vi "GdsLanguage_UpdateAllControlsOnVI.vi"(0 "Viref/PathToUpdate(If Empty Uses the caller)":variant, 2 "MatchControlLabelName":string="^_", 5 "error in (no error)":errorcluster, 7 "CreateLanguageFile(Use this to create a languageFile)":bool) -> (13 "AllLanguageFile":string, 19 "error out":errorcluster)   [LabVIEW 2020]
doc: "Returns a translated string based on the value of the StringID parameter."
panel:
  out "OnlyNew":string
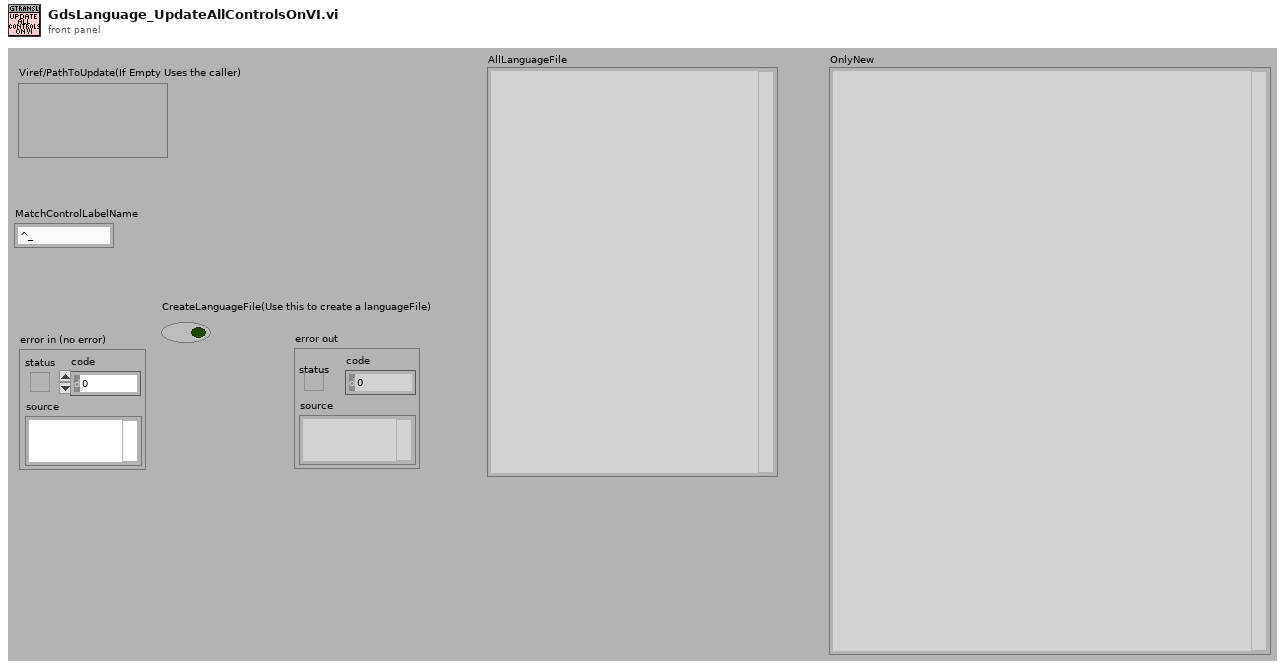
[diagram p1: front panel]
types:
  T1 = cluster{"ViRef":refnum<vi>, "Controls":refnum<vi>[], "RefCreated":bool}
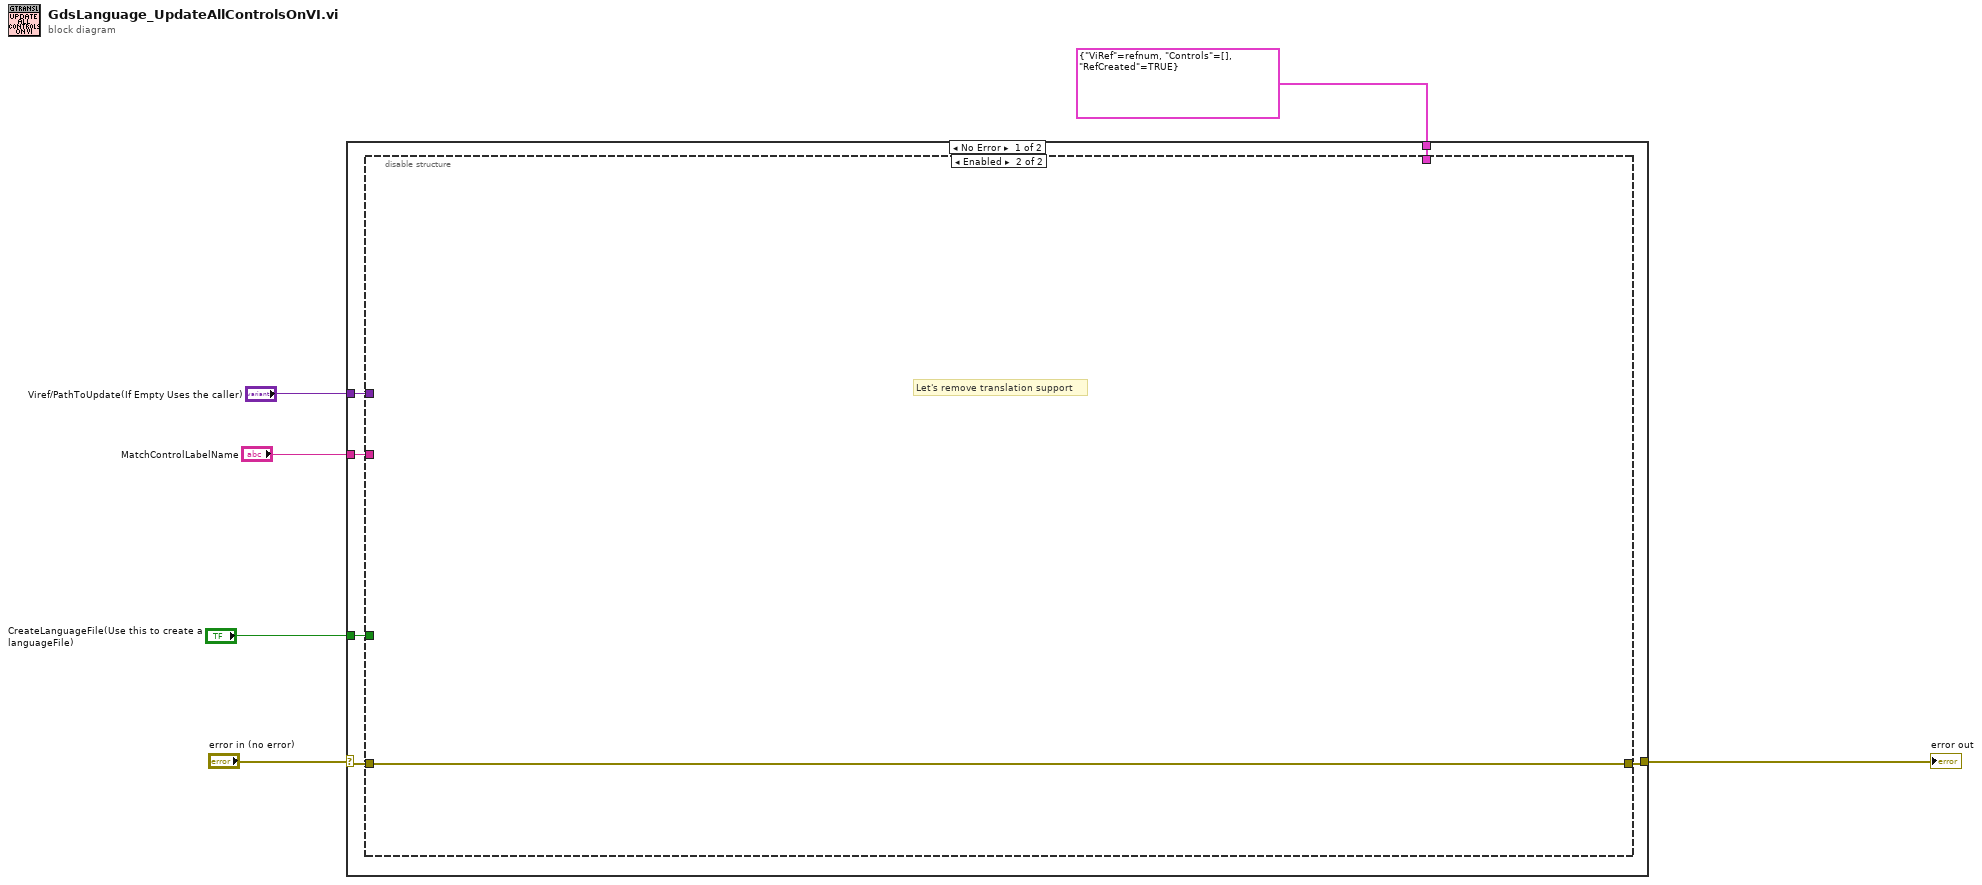
[diagram p0: block diagram]
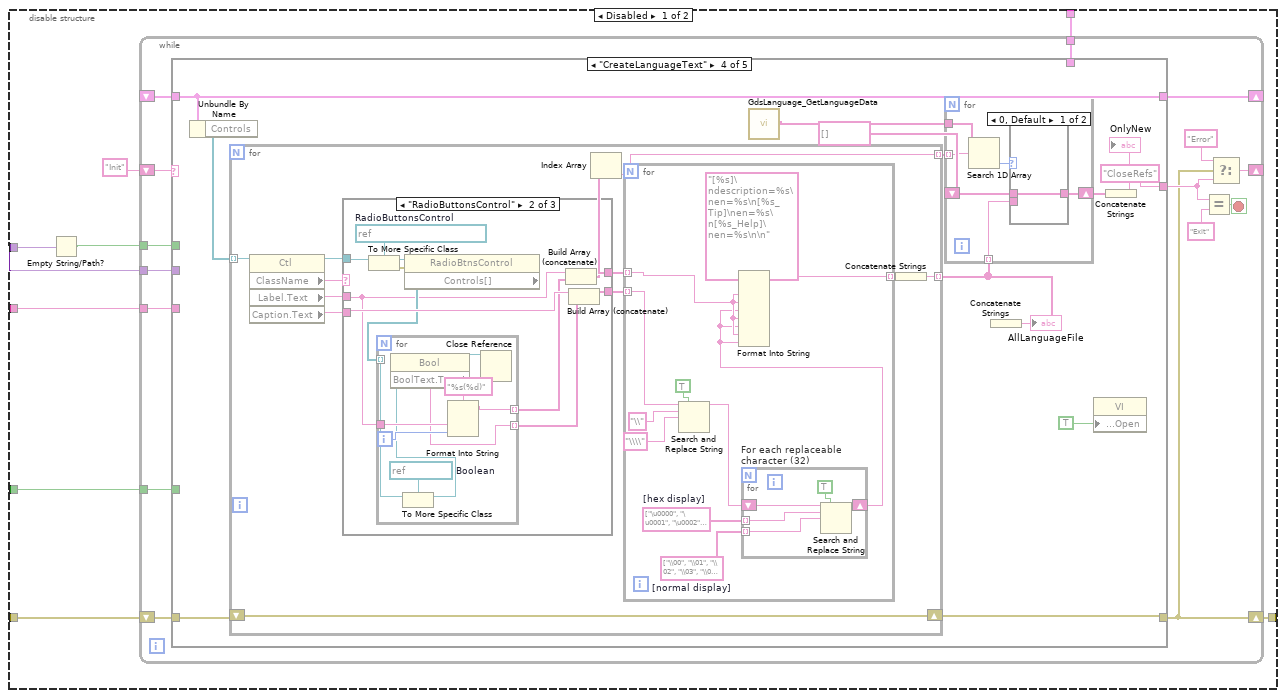
[diagram p2: hidden frame]
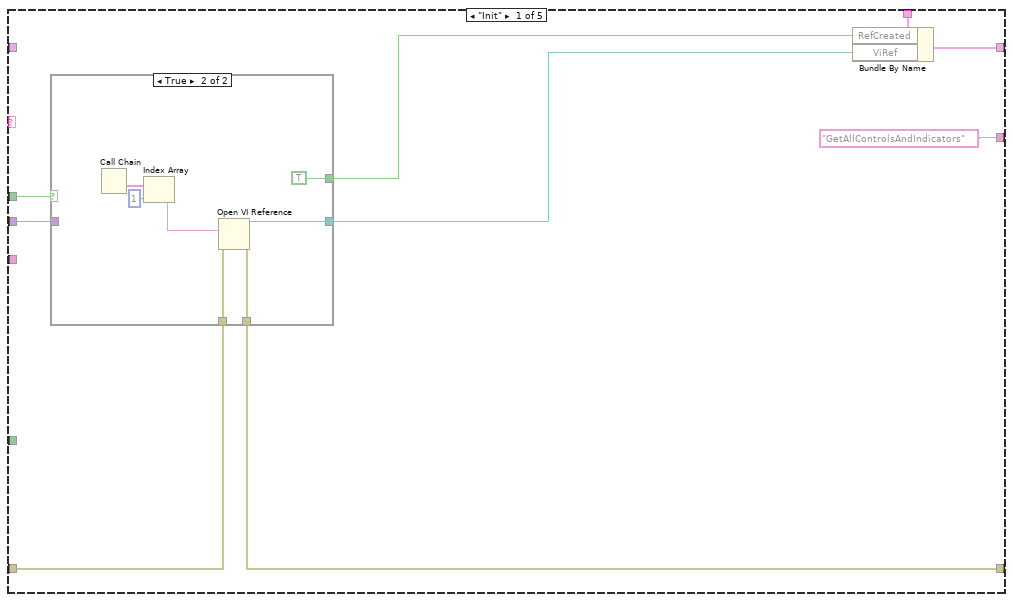
[diagram p3: hidden frame]
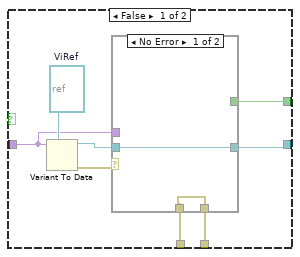
[diagram p4: hidden frame]
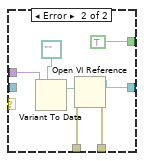
[diagram p5: hidden frame]
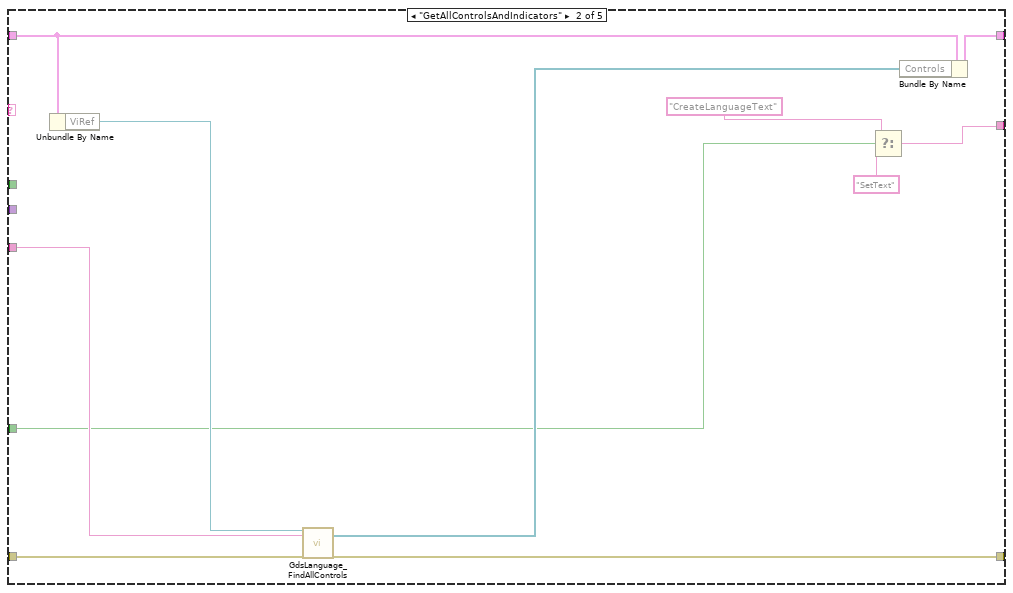
[diagram p6: hidden frame]
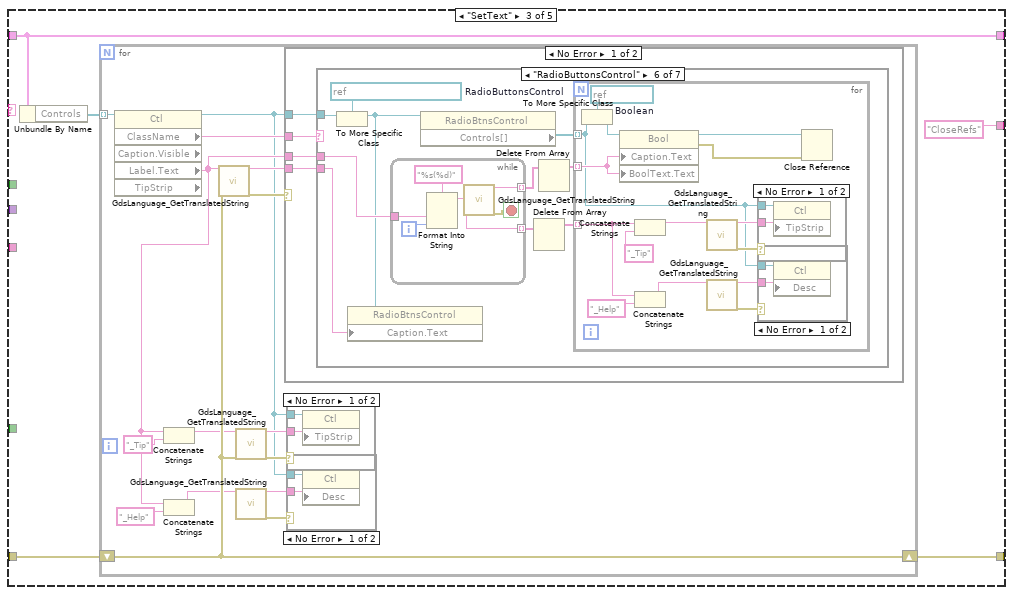
[diagram p7: hidden frame]
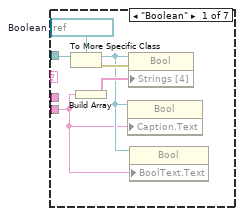
[diagram p10: hidden frame]
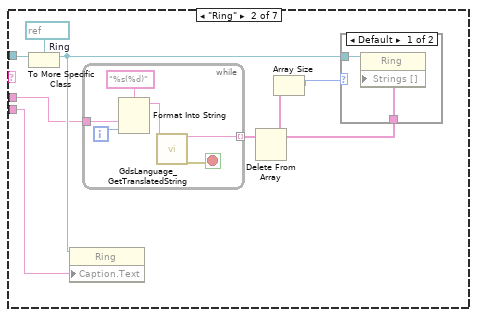
[diagram p11: hidden frame]
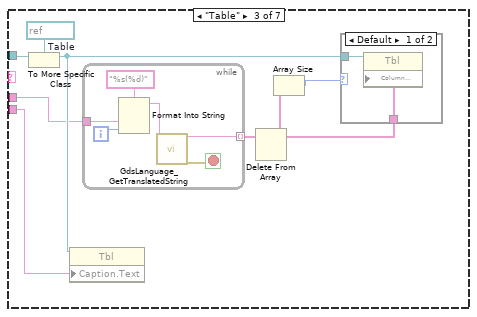
[diagram p13: hidden frame]
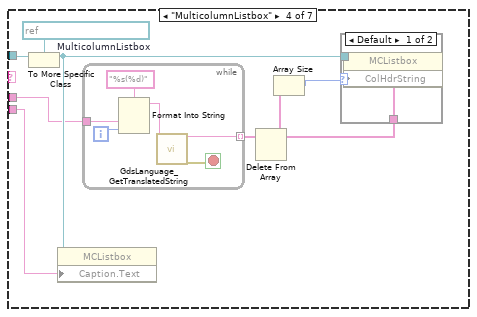
[diagram p15: hidden frame]
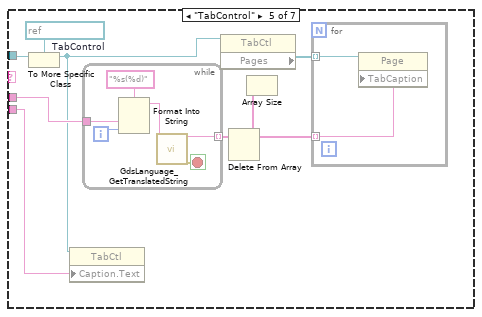
[diagram p17: hidden frame]
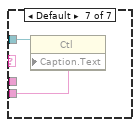
[diagram p20: hidden frame]
diagram:
  n1 = case shown="No Error" "error in (no error)" {
    selector: "error in (no error)" -> [w12 w315]
    tunnel: [w9 w315] -> w5
    tunnel: "Viref/PathToUpdate(If Empty Uses the caller)" -> [w8 _]
    tunnel: "CreateLanguageFile(Use this to create a languageFile)" -> [w7 _]
    tunnel: T1 {"ViRef"=refnum, "Controls"=[], "RefCreated"=TRUE} -> [w11 _]
    tunnel: "MatchControlLabelName" -> [w10 _]
    frame No Error {
      n2 = disable-structure shown="Enabled" {
        disable-tunnel: w12 -> [w19 w314]
        disable-tunnel: w11 -> [w18 _]
        disable-tunnel: w10 -> [w17 _]
        disable-tunnel: [w16 w314] -> w9
        disable-tunnel: w8 -> [w15 _]
        disable-tunnel: w7 -> [w13 _]
        frame Disabled {
          n3 = Empty String/Path?(string/path=w15) -> (empty?=w14:bool)
          n4 = while {
            shift-right: [w28] -> w16
            shift-left: w19 -> [w35]
            shift-right: [w33] -> _
            shift-left: "Init" -> [w34]
            shift-right: [w27] -> _
            shift-left: _ -> [w26]
            tunnel: w14 -> [w25]
            tunnel: w18 -> [w24]
            tunnel: w15 -> [w23]
            tunnel: w17 -> [w22]
            tunnel: w13 -> [w21]
            stop <- w32 stop-if-true
            n5 = case shown="\"CreateLanguageText\"" w34 {
              tunnel: w35 -> [w38 w79 w84 w227 w305]
              tunnel: [w37 w76 w82 w215 w298] -> w28
              tunnel: ["GetAllControlsAndIndicators" w70 "CloseRefs" "CloseRefs" "Exit"] -> w29
              tunnel: [w39 w73 w80 w224 w301] -> w27
              tunnel: w26 -> [_ w75 w80 w224 w301]
              tunnel: w25 -> [w43 _ _ _ _]
              tunnel: w24 -> [w42 _ _ _ _]
              tunnel: w23 -> [w40 _ _ _ _]
              tunnel: w22 -> [_ w78 _ _ _]
              tunnel: w21 -> [_ w72 _ _ w299]
              frame "Init" {
                n6 = case shown="True" w43 {
                  tunnel: w38 -> [w51 w65]
                  tunnel: [w47 w64] -> w41
                  tunnel: w40 -> [w46 _]
                  tunnel: [w50 w63] -> w37
                  tunnel: [w45 TRUE] -> w36
                  frame False {
                    w52 = refnum<vi> refnum  # ViRef
                    n7 = Variant To Data(type=w52, Variant=w46) -> (data=w48:refnum<vi>, error out=w49:errorcluster)  [unwired: 1 in]
                    n8 = case shown="No Error" w49 {
                      tunnel: w51 -> [w53 w61]
                      tunnel: [w53 w60] -> w50
                      tunnel: [w54 w56] -> w47
                      tunnel: w48 -> [w54 _]
                      tunnel: w46 -> [_ w59]
                      tunnel: [_ TRUE] -> w45
                      frame No Error {
                      }
                      frame Error {
                        n9 = Variant To Data(type=path "", Variant=w59) -> (data=w57:path)  [unwired: 1 in, 1 out]
                        n10 = Open VI Reference(vi path=w57, error in (no error)=w61) -> (vi reference=w56:refnum<vi>, error out=w60:errorcluster)  [unwired: 4 in]
                      }
                    }
                  }
                  frame True {
                    n11 = Call Chain() -> (call chain=w68:string[])
                    n12 = Index Array(array=w68, index=1) -> (element=w66:string)
                    n13 = Open VI Reference(vi path=w66, error in (no error)=w65) -> (vi reference=w64:refnum<vi>, error out=w63:errorcluster)  [unwired: 4 in]
                  }
                }
                n14 = Bundle By Name(cluster=w42, "RefCreated"=w36, "ViRef"=w41) -> (w39:T1)
              }
              frame "GetAllControlsAndIndicators" {
                n15 = Unbundle By Name(w75) -> ("ViRef"=w77:refnum<vi>)
                n16 = call <resource>:"GdsLanguage_FindAllControls.vi"("ViRef"=w77, "LabelMatchPattern"=w78, "error in (no error)"=w79) -> ("ControlsFound"=w74:refnum<vi>[], "error out"=w76:errorcluster)  [unwired: 15 in]
                n17 = Select(t="CreateLanguageText", s=w72, f="SetText") -> (s? t:f=w70:string)
                n18 = Bundle By Name(cluster=w75, "Controls"=w74) -> (w73:T1)
              }
              frame "SetText" {
                n19 = Unbundle By Name(w80) -> ("Controls"=w83:refnum<vi>[])
                n20 = for {
                  shift-right: [w95] -> w82
                  shift-left: w84 -> [w95]
                  tunnel: w83 -> [w99] mode=indexing
                  n21 = property class="Ctl" props=["ClassName", "Caption", "Visible", "Label", "Text", "TipStrip"](reference=w99) -> (reference out=w86:refnum<vi>, "ClassName"=w98:string, "Label.Text"=w89:string)  [unwired: 1 in, 3 out]
                  n22 = Concatenate Strings(w89, "_Tip" ("string")) -> (w92:string)
                  n23 = Concatenate Strings(w89, "_Help" ("string")) -> (w85:string)
                  n24 = call <resource>:"GdsLanguage_GetTranslatedString.vi"("StringID(s)"=w89, "error in (no error)"=w95) -> ("FirstStringOut"=w96:string, "error out"=w97:errorcluster)  [unwired: 14 in, 2 out]
                  n25 = call <resource>:"GdsLanguage_GetTranslatedString.vi"("StringID(s)"=w92, "error in (no error)"=w95) -> ("FirstStringOut"=w91:string, "error out"=w94:errorcluster)  [unwired: 14 in, 2 out]
                  n26 = call <resource>:"GdsLanguage_GetTranslatedString.vi"("StringID(s)"=w85) -> ("FirstStringOut"=w88:string, "error out"=w87:errorcluster)  [unwired: 15 in, 2 out]
                  n27 = case shown="No Error" w97 {
                    tunnel: w98 -> [w107 _]
                    tunnel: w86 -> [w105 _]
                    tunnel: w96 -> [w106 _]
                    tunnel: w89 -> [w104 _]
                    frame No Error {
                      n28 = case shown="\"RadioButtonsControl\"" w107 {
                        tunnel: w105 -> [w113 w121 w137 w153 w169 w187 w214]
                        tunnel: w106 -> [w108 w118 w134 w150 w167 w186 w213]
                        tunnel: w104 -> [_ w117 w133 w149 w166 w185 _]
                        frame "Boolean" {
                          w112 = refnum<vi> refnum  # Boolean
                          n29 = To More Specific Class(target class=w112, reference=w113) -> (specific class reference=w109:refnum<vi>, error out=w111:errorcluster)  [unwired: 1 in]
                          n30 = Build Array(w108) -> (w110:string[])
                          n31 = property class="Bool"(reference=w109, "Caption.Text"=w108) -> ()  [unwired: 1 in, 2 out]
                          n32 = property class="Bool"(reference=w109, error in=w111, "Strings [4]"=w110) -> ()  [unwired: 2 out]
                          n33 = property class="Bool"(reference=w109, "BoolText.Text"=w108) -> ()  [unwired: 1 in, 2 out]
                        }
                        frame "Ring" {
                          w120 = refnum<vi> refnum  # Ring
                          n34 = To More Specific Class(target class=w120, reference=w121) -> (specific class reference=w119:refnum<vi>)  [unwired: 1 in, 1 out]
                          n35 = property class="Ring"(reference=w119, "Caption.Text"=w118) -> ()  [unwired: 1 in, 2 out]
                          n36 = while {
                            tunnel: w117 -> [w126]
                            tunnel: [w122] -> w116 mode=indexing
                            i -> [w125]
                            stop <- w123 stop-if-true
                            n37 = Format Into String(format string="%s(%d)", w126, w125) -> (resulting string=w124:string)  [unwired: 2 in, 1 out]
                            n38 = call <resource>:"GdsLanguage_GetTranslatedString.vi"("StringID(s)"=w124) -> ("FirstStringOut"=w122:string, "error out"=w123:errorcluster)  [unwired: 15 in, 2 out]
                          }
                          n39 = Delete From Array(array=w116) -> (array with subset deleted=w114:string[])  [unwired: 2 in, 1 out]
                          n40 = Array Size(array=w114) -> (size(s)=w115:i32)
                          n41 = case shown="Default" w115 {
                            tunnel: w119 -> [w129 _]
                            tunnel: w114 -> [w128 _]
                            frame Default {
                              n42 = property class="Ring"(reference=w129, "Strings []"=w128) -> ()  [unwired: 1 in, 2 out]
                            }
                            frame 0 {
                            }
                          }
                        }
                        frame "Table" {
                          w136 = refnum<vi> refnum  # Table
                          n43 = To More Specific Class(target class=w136, reference=w137) -> (specific class reference=w135:refnum<vi>)  [unwired: 1 in, 1 out]
                          n44 = property class="Tbl"(reference=w135, "Caption.Text"=w134) -> ()  [unwired: 1 in, 2 out]
                          n45 = while {
                            tunnel: w133 -> [w142]
                            tunnel: [w138] -> w132 mode=indexing
                            i -> [w141]
                            stop <- w139 stop-if-true
                            n46 = Format Into String(format string="%s(%d)", w142, w141) -> (resulting string=w140:string)  [unwired: 2 in, 1 out]
                            n47 = call <resource>:"GdsLanguage_GetTranslatedString.vi"("StringID(s)"=w140) -> ("FirstStringOut"=w138:string, "error out"=w139:errorcluster)  [unwired: 15 in, 2 out]
                          }
                          n48 = Delete From Array(array=w132) -> (array with subset deleted=w130:string[])  [unwired: 2 in, 1 out]
                          n49 = Array Size(array=w130) -> (size(s)=w131:i32)
                          n50 = case shown="Default" w131 {
                            tunnel: w135 -> [w145 _]
                            tunnel: w130 -> [w144 _]
                            frame Default {
                              n51 = property class="Tbl"(reference=w145, "Column Headers[]"=w144) -> ()  [unwired: 1 in, 2 out]
                            }
                            frame 0 {
                            }
                          }
                        }
                        frame "MulticolumnListbox" {
                          w152 = refnum<vi> refnum  # MulticolumnListbox
                          n52 = To More Specific Class(target class=w152, reference=w153) -> (specific class reference=w151:refnum<vi>)  [unwired: 1 in, 1 out]
                          n53 = property class="MCListbox"(reference=w151, "Caption.Text"=w150) -> ()  [unwired: 1 in, 2 out]
                          n54 = while {
                            tunnel: w149 -> [w158]
                            tunnel: [w154] -> w148 mode=indexing
                            i -> [w157]
                            stop <- w155 stop-if-true
                            n55 = Format Into String(format string="%s(%d)", w158, w157) -> (resulting string=w156:string)  [unwired: 2 in, 1 out]
                            n56 = call <resource>:"GdsLanguage_GetTranslatedString.vi"("StringID(s)"=w156) -> ("FirstStringOut"=w154:string, "error out"=w155:errorcluster)  [unwired: 15 in, 2 out]
                          }
                          n57 = Delete From Array(array=w148) -> (array with subset deleted=w146:string[])  [unwired: 2 in, 1 out]
                          n58 = Array Size(array=w146) -> (size(s)=w147:i32)
                          n59 = case shown="Default" w147 {
                            tunnel: w151 -> [w161 _]
                            tunnel: w146 -> [w160 _]
                            frame Default {
                              n60 = property class="MCListbox"(reference=w161, "ColHdrString"=w160) -> ()  [unwired: 1 in, 2 out]
                            }
                            frame 0 {
                            }
                          }
                        }
                        frame "TabControl" {
                          w168 = refnum<vi> refnum  # TabControl
                          n61 = To More Specific Class(target class=w168, reference=w169) -> (specific class reference=w163:refnum<vi>)  [unwired: 1 in, 1 out]
                          n62 = property class="TabCtl"(reference=w163, "Caption.Text"=w167) -> ()  [unwired: 1 in, 2 out]
                          n63 = while {
                            tunnel: w166 -> [w176]
                            tunnel: [w172] -> w165 mode=indexing
                            i -> [w175]
                            stop <- w173 stop-if-true
                            n64 = Format Into String(format string="%s(%d)", w176, w175) -> (resulting string=w174:string)  [unwired: 2 in, 1 out]
                            n65 = call <resource>:"GdsLanguage_GetTranslatedString.vi"("StringID(s)"=w174) -> ("FirstStringOut"=w172:string, "error out"=w173:errorcluster)  [unwired: 15 in, 2 out]
                          }
                          n66 = property class="TabCtl"(reference=w163) -> ("Pages"=w162:refnum<vi>[])  [unwired: 1 in, 2 out]
                          n67 = Delete From Array(array=w165) -> (array with subset deleted=w164:string[])  [unwired: 2 in, 1 out]
                          n68 = Array Size(array=w164) -> ()  [unwired: 1 out]
                          n69 = for {
                            tunnel: w164 -> [w171] mode=indexing
                            tunnel: w162 -> [w170] mode=indexing
                            n70 = property class="Page"(reference=w170, "TabCaption"=w171) -> ()  [unwired: 1 in, 2 out]
                          }
                        }
                        frame "RadioButtonsControl" {
                          w180 = refnum<vi> refnum  # RadioButtonsControl
                          n71 = To More Specific Class(target class=w180, reference=w187) -> (specific class reference=w182:refnum<vi>)  [unwired: 1 in, 1 out]
                          n72 = property class="RadioBtnsControl"(reference=w182, "Caption.Text"=w186) -> ()  [unwired: 1 in, 2 out]
                          n73 = while {
                            tunnel: w185 -> [w211]
                            tunnel: [w208] -> w184 mode=indexing
                            tunnel: [w207] -> w179 mode=indexing
                            i -> [w210]
                            stop <- w209 stop-if-true
                            n74 = Format Into String(format string="%s(%d)", w211, w210) -> (resulting string=w207:string)  [unwired: 2 in, 1 out]
                            n75 = call <resource>:"GdsLanguage_GetTranslatedString.vi"("StringID(s)"=w207) -> ("FirstStringOut"=w208:string, "error out"=w209:errorcluster)  [unwired: 15 in, 2 out]
                          }
                          n76 = property class="RadioBtnsControl"(reference=w182) -> ("Controls[]"=w181:refnum<vi>[])  [unwired: 1 in, 2 out]
                          n77 = Delete From Array(array=w179) -> (array with subset deleted=w178:string[])  [unwired: 2 in, 1 out]
                          n78 = Delete From Array(array=w184) -> (array with subset deleted=w183:string[])  [unwired: 2 in, 1 out]
                          n79 = for {
                            tunnel: w183 -> [w196] mode=indexing
                            tunnel: w181 -> [w189] mode=indexing
                            tunnel: w178 -> [w188] mode=indexing
                            w200 = refnum<vi> refnum  # Boolean
                            n80 = To More Specific Class(target class=w200, reference=w189) -> (specific class reference=w199:refnum<vi>)  [unwired: 1 in, 1 out]
                            n81 = property class="Bool"(reference=w199, "Caption.Text"=w196, "BoolText.Text"=w196) -> (reference out=w201:refnum<vi>, error out=w202:errorcluster)  [unwired: 1 in]
                            n82 = Concatenate Strings(w188, "_Tip" ("string")) -> (w191:string)
                            n83 = Concatenate Strings(w188, "_Help" ("string")) -> (w190:string)
                            n84 = call <resource>:"GdsLanguage_GetTranslatedString.vi"("StringID(s)"=w191) -> ("FirstStringOut"=w193:string, "error out"=w192:errorcluster)  [unwired: 15 in, 2 out]
                            n85 = call <resource>:"GdsLanguage_GetTranslatedString.vi"("StringID(s)"=w190) -> ("FirstStringOut"=w194:string, "error out"=w195:errorcluster)  [unwired: 15 in, 2 out]
                            n86 = case shown="No Error" w192 {
                              tunnel: w193 -> [w206 _]
                              tunnel: w189 -> [w205 _]
                              frame No Error {
                                n87 = property class="Ctl"(reference=w205, "TipStrip"=w206) -> ()  [unwired: 1 in, 2 out]
                              }
                              frame Error {
                              }
                            }
                            n88 = case shown="No Error" w195 {
                              tunnel: w194 -> [w204 _]
                              tunnel: w189 -> [w203 _]
                              frame No Error {
                                n89 = property class="Ctl"(reference=w203, "Desc"=w204) -> ()  [unwired: 1 in, 2 out]
                              }
                              frame Error {
                              }
                            }
                            n90 = Close Reference(reference=w201, error in (no error)=w202) -> ()  [unwired: 1 out]
                          }
                        }
                        frame Default {
                          n91 = property class="Ctl"(reference=w214, "Caption.Text"=w213) -> ()  [unwired: 1 in, 2 out]
                        }
                      }
                    }
                    frame Error {
                    }
                  }
                  n92 = case shown="No Error" w94 {
                    tunnel: w91 -> [w103 _]
                    tunnel: w86 -> [w102 _]
                    frame No Error {
                      n93 = property class="Ctl"(reference=w102, "TipStrip"=w103) -> ()  [unwired: 1 in, 2 out]
                    }
                    frame Error {
                    }
                  }
                  n94 = case shown="No Error" w87 {
                    tunnel: w88 -> [w101 _]
                    tunnel: w86 -> [w100 _]
                    frame No Error {
                      n95 = property class="Ctl"(reference=w100, "Desc"=w101) -> ()  [unwired: 1 in, 2 out]
                    }
                    frame Error {
                    }
                  }
                }
              }
              frame "CreateLanguageText" {
                n96 = Unbundle By Name(w224) -> ("Controls"=w226:refnum<vi>[])
                n97 = for {
                  shift-right: [w245] -> w215
                  shift-left: w227 -> [w245]
                  tunnel: w226 -> [w248] mode=indexing
                  tunnel: [w240] -> w219 mode=indexing
                  tunnel: [w238] -> w221 mode=indexing
                  n98 = property class="Ctl"(reference=w248) -> (reference out=w246:refnum<vi>, "ClassName"=w247:string, "Label.Text"=w241:string, "Caption.Text"=w244:string)  [unwired: 1 in, 1 out]
                  n99 = case shown="\"RadioButtonsControl\"" w247 {
                    tunnel: w246 -> [w273 w284 _]
                    tunnel: [w267 w279 w296] -> w242
                    tunnel: w244 -> [_ w278 w297]
                    tunnel: w241 -> [w265 w274 w295]
                    tunnel: [w266 w280 w294] -> w239
                    frame "Boolean" {
                      w272 = refnum<vi> refnum  # Boolean
                      n100 = To More Specific Class(target class=w272, reference=w273) -> (specific class reference=w271:refnum<vi>, error out=w270:errorcluster)  [unwired: 1 in]
                      n101 = property class="Bool"(reference=w271, error in=w270) -> ("Strings [4]"=w269:string[])  [unwired: 2 out]
                      n102 = Index Array(array=w269) -> (element=w268:string)  [unwired: 1 in]
                      n103 = Build Array(w265) -> (w266:string[])
                      n104 = Build Array(w268) -> (w267:string[])
                    }
                    frame "RadioButtonsControl" {
                      w283 = refnum<vi> refnum  # RadioButtonsControl
                      n105 = To More Specific Class(target class=w283, reference=w284) -> (specific class reference=w282:refnum<vi>, error out=w281:errorcluster)  [unwired: 1 in]
                      n106 = property class="RadioBtnsControl"(reference=w282, error in=w281) -> ("Controls[]"=w277:refnum<vi>[])  [unwired: 2 out]
                      n107 = for {
                        tunnel: w277 -> [w286] mode=indexing
                        tunnel: [w290] -> w276 mode=indexing
                        tunnel: [w289] -> w275 mode=indexing
                        tunnel: w274 -> [w291]
                        i -> [w292]
                        w287 = refnum<vi> refnum  # Boolean
                        n108 = To More Specific Class(target class=w287, reference=w286) -> (specific class reference=w285:refnum<vi>)  [unwired: 1 in, 1 out]
                        n109 = property class="Bool"(reference=w285) -> (reference out=w288:refnum<vi>, "BoolText.Text"=w289:string)  [unwired: 1 in, 1 out]
                        n110 = Format Into String(format string="%s(%d)", w291, w292) -> (resulting string=w290:string)  [unwired: 2 in, 1 out]
                        n111 = Close Reference(reference=w288) -> ()  [unwired: 1 in, 1 out]
                      }
                      n112 = Build Array (concatenate)(w274, w276) -> (w280:string[])
                      n113 = Build Array (concatenate)(w278, w275) -> (w279:string[])
                    }
                    frame Default {
                      n114 = Build Array(w295) -> (w294:string[])
                      n115 = Build Array(w297) -> (w296:string[])
                    }
                  }
                  n116 = Index Array(array=w239) -> (element=w238:string)  [unwired: 1 in]
                  n117 = for {
                    tunnel: [w258] -> w243 mode=indexing
                    tunnel: w242 -> [w253] mode=indexing
                    tunnel: w239 -> [w257] mode=indexing
                    w249 = string[] ["\u0000", "\u0001", "\u0002", "\u0003", "\u0004", "\u0005", "\u0006", "\u0007", "\b", "\t", "\n", "\u000b", "\f", "\r", "\u000e", "\u000f", "\u0010", "\u0011", "\u0012", "\u0013", "\u0014", "\u0015", "\u0016", "\u0017", "\u0018", "\u0019", "\u001a", "\u001b", "\u001c", "\u001d", "\u001e", "\u001f"]  # [hex display]
                    w252 = string[] ["\\00", "\\01", "\\02", "\\03", "\\04", "\\05", "\\06", "\\07", "\\08", "\\09", "\\0A", "\\0B", "\\0C", "\\0D", "\\0E", "\\0F", "\\10", "\\11", "\\12", "\\13", "\\14", "\\15", "\\16", "\\17", "\\18", "\\19", "\\1A", "\\1B", "\\1C", "\\1D", "\\1E", "\\1F"]  # [normal display]
                    n118 = Search and Replace String(replace all?=TRUE ("replace all? (F)"), input string=w253, search string="\\" ("regular expression"), replace string="\\\\") -> (result string=w251:string)  [unwired: 4 in, 3 out]
                    n119 = for "For each replaceable character (32)" {
                      shift-right: [w263] -> w250
                      shift-left: w251 -> [w264]
                      tunnel: w252 -> [w262] mode=indexing
                      tunnel: w249 -> [w261] mode=indexing
                      n120 = Search and Replace String(replace all?=TRUE ("replace all? (F)"), input string=w264, search string=w261, replace string=w262) -> (result string=w263:string)  [unwired: 4 in, 3 out]
                    }
                    n121 = Format Into String(format string="[%s]\ndescription=%s\nen=%s\n[%s_Tip]\nen=%s\n[%s_Help]\nen=%s\n\n", w257, w257, w250, w257, w250, w257, w250) -> (resulting string=w258:string)  [unwired: 2 in, 1 out]
                  }
                  n122 = Concatenate Strings(w243) -> (w240:string)
                }
                n123 = call <resource>:"GdsLanguage_GetLanguageData.vi"() -> ("StringIDArray"=w220:string[])  [unwired: 15 in, 4 out]
                n124 = for {
                  tunnel: w221 -> [w233] mode=indexing
                  tunnel: w220 -> [w232]
                  shift-right: [w229] -> w218
                  shift-left: string[] [] -> [w230]
                  tunnel: w219 -> [w228] mode=indexing
                  n125 = Search 1D Array(1D array=w232, element=w233) -> (index of element=w231:i32)  [unwired: 1 in]
                  n126 = case shown="0, Default" w231 {
                    tunnel: w230 -> [w234 w237]
                    tunnel: [w234 w236] -> w229
                    tunnel: w228 -> [_ w235]
                    frame 0, Default {
                    }
                    frame -1 {
                      n127 = Build Array (concatenate)(w237, w235) -> (w236:string[])
                    }
                  }
                }
                n128 = Concatenate Strings(w219) -> (→"AllLanguageFile":string)
                n129 = property class="VI"("Front Panel.Open"=TRUE ("Front Panel Window:Open")) -> ()  [unwired: 2 in, 2 out]
                n130 = Concatenate Strings(w218) -> (→"OnlyNew":string)
              }
              frame "CloseRefs", "Error", Default {
                n131 = Unbundle By Name(w301) -> ("ViRef"=w303:refnum<vi>, "RefCreated"=w300:bool, "Controls"=w306:refnum<vi>[])
                n132 = for {
                  tunnel: w306 -> [w313] mode=indexing
                  shift-right: [w311] -> w304
                  shift-left: w305 -> [w312]
                  n133 = Close Reference(reference=w313, error in (no error)=w312) -> (error out=w311:errorcluster)
                }
                n134 = case shown="True" w300 {
                  tunnel: w304 -> [w307 w310]
                  tunnel: [w307 w309] -> w298
                  tunnel: w303 -> [_ w308]
                  frame False {
                  }
                  frame True {
                    n135 = Close Reference(reference=w308, error in (no error)=w310) -> (error out=w309:errorcluster)
                  }
                }
                n136 = case shown="True" w299 {
                  tunnel: w298 -> [_ _]
                  frame False {
                  }
                  frame True {
                    n137 = Stop() -> ()  [unwired: 1 in]
                  }
                }
              }
            }
            n138 = Equal?(x=w29, y="Exit") -> (x = y?=w32:bool)
            n139 = Select(t="Error", s=w28, f=w29) -> (s? t:f=w33:string)
          }
        }
        frame Enabled {
          # "Let's remove translation support"
        }
      }
    }
    frame Error {
    }
  }
  "error out" <- w5
